vi "FIU card.vi"(8 "error in (no error)":errorcluster, 11 "Node Ptr":T3 format="%.0x") -> (0 "error out":errorcluster)   [LabVIEW 2013, in "SLSC configuration System Explorer.lvlib"]
uses:
  SLSC configuration System Explorer.lvlib
  <vilib>/NI Veristand/Custom Device API/Custom Device Item Ref.ctl
  Shared/Card Postion.ctl
  Shared/Constants.vi
  <vilib>/NI Veristand/Custom Device API/Get Item Property (U16).vi
  <vilib>/NI Veristand/Custom Device API/Set Item Property (Variant).vi
  <vilib>/NI Veristand/Custom Device API/Custom Device API.lvlib
  Shared/SLSC configuration Shared.lvlib
panel:
  in  "Card Position":T1
  in  "Fault 8":T2(ring)
  in  "Fault 7":T2(ring)
  in  "Fault 6":T2(ring)
  in  "Fault 5":T2(ring)
  in  "Fault 4":T2(ring)
  in  "Fault 3":T2(ring)
  in  "Fault 2":T2(ring)
  in  "Header 2":cluster{"Section Name":string}={"Section Name"="FIU Initial Configuration"}
  in  "Fault 1":T2(ring)
  in  "Header":cluster{"Section Name":string}={"Section Name"="FIU Card Settings"}
  in  "Description":string
  in  "Name":string
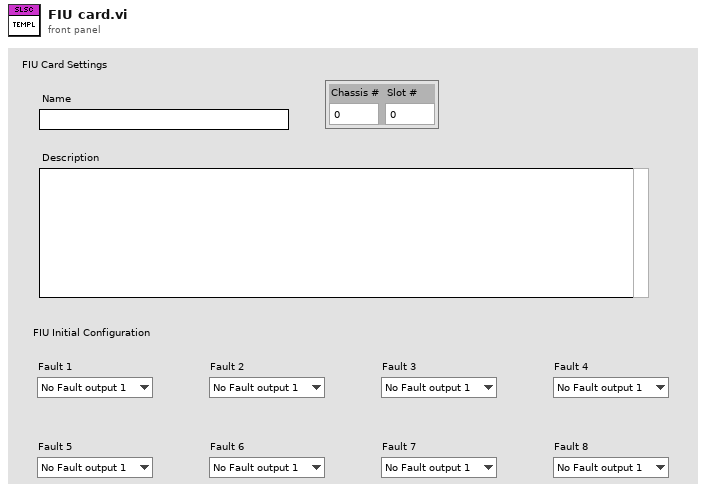
[diagram p1: front panel]
types:
  T1 = typedef "SLSC configuration Shared.lvlib/Card Postion.ctl" = cluster{"Chassis #":u8, "Slot #":u8}
  T2 = enum16{"No Fault output 1", "Open Ckt 100Hz", "Ground 100Hz", "Open Circuit", "Ground", "Rail 1", "Rail 2", "No Fault output 2"}
  T3 = typedef "Custom Device API.lvlib/Custom Device Item Ref.ctl" = u64
  T4 = typedef "Custom Device API.lvlib/Custom Device Commands.ctl" = enum16{"Default", "Item renamed", "Shutdown", "Dynamic button pressed"}
  T5 = typedef "Custom Device API.lvlib/Custom Device Item Info.ctl" = cluster{"Name":string, "Is Channel":bool, "GUID":string, "Is Waveform":bool}
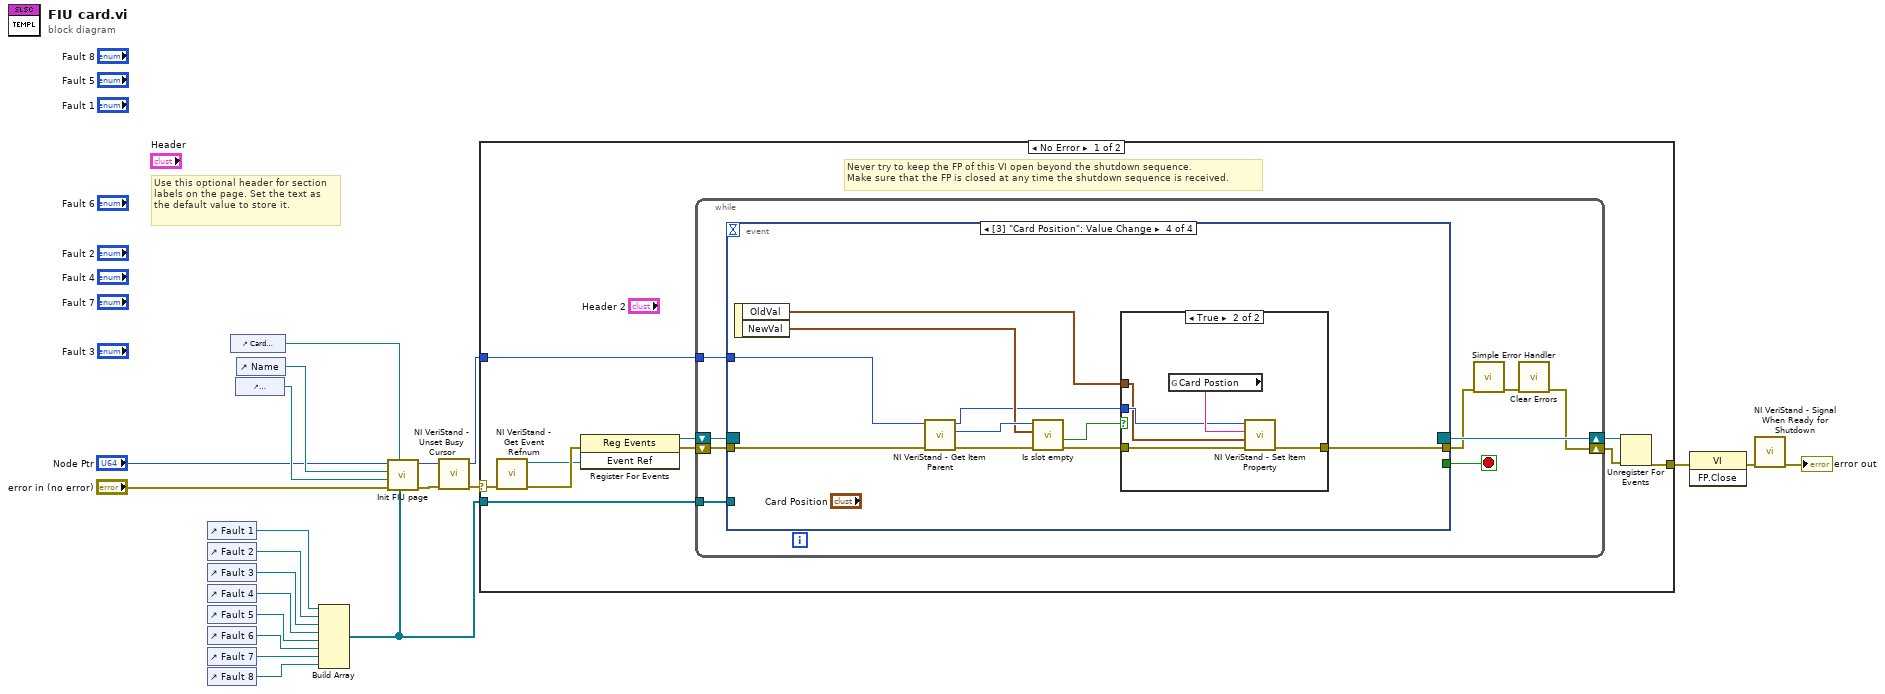
[diagram p0: block diagram]
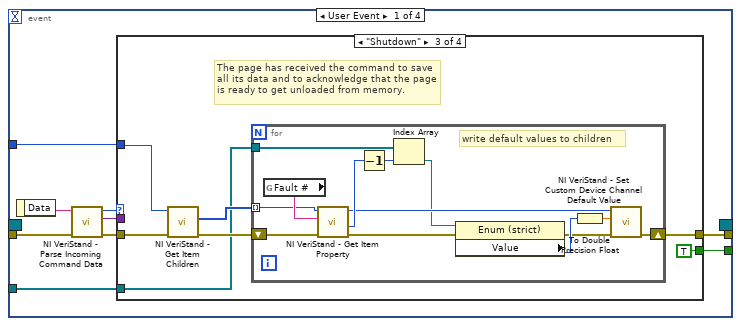
[diagram p2: hidden frame]
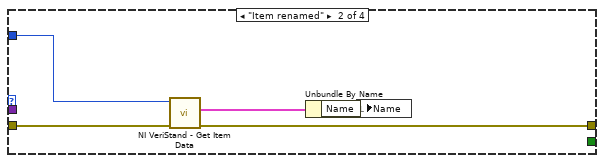
[diagram p4: hidden frame]
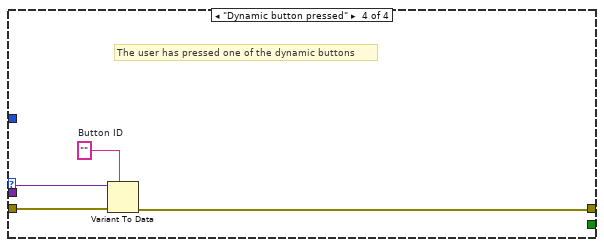
[diagram p5: hidden frame]
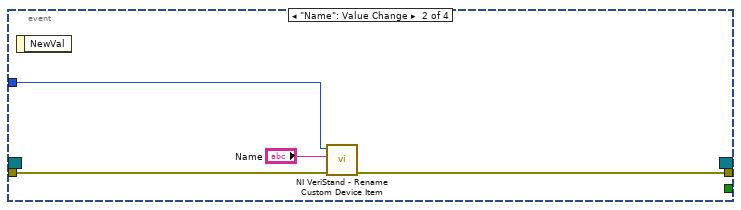
[diagram p6: hidden frame]
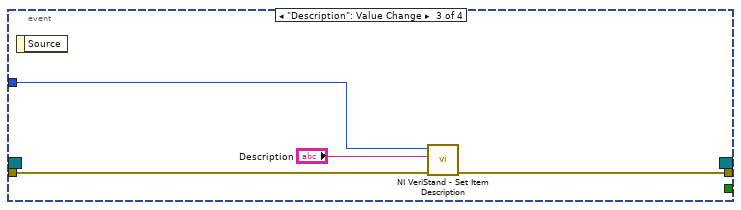
[diagram p7: hidden frame]
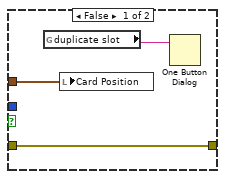
[diagram p8: hidden frame]
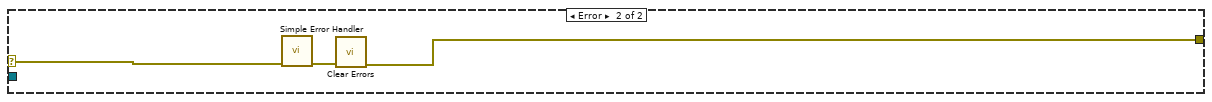
[diagram p9: hidden frame]
diagram:
  # "Use this optional header for section labels on the page. Set the text as the default value to store it."
  n1 = control-ref of="Fault 1"() -> (w13:refnum<vi>)
  n2 = control-ref of="Fault 2"() -> (w12:refnum<vi>)
  n3 = control-ref of="Fault 3"() -> (w11:refnum<vi>)
  n4 = control-ref of="Fault 4"() -> (w10:refnum<vi>)
  n5 = control-ref of="Fault 5"() -> (w9:refnum<vi>)
  n6 = control-ref of="Fault 6"() -> (w8:refnum<vi>)
  n7 = control-ref of="Fault 7"() -> (w7:refnum<vi>)
  n8 = control-ref of="Fault 8"() -> (w6:refnum<vi>)
  n9 = control-ref of="Card Position"() -> (w1:refnum<vi>)
  n10 = control-ref of="Description"() -> (w4:refnum<vi>)
  n11 = control-ref of="Name"() -> (w5:refnum<vi>)
  n12 = Build Array(w13, w12, w11, w10, w9, w8, w7, w6) -> (w2:refnum<vi>[])
  n13 = call "Init FIU page.vi"("Fault controls"=w2, "Card Position"=w1, "error in (no error)"="error in (no error)", "Description"=w4, "Name"=w5, "Node Ptr"="Node Ptr") -> ("error out"=w17:errorcluster, "Node Ptr out"=w14:T3)  [unwired: 4 in]
  n14 = call <vilib>:"NI VeriStand - Unset Busy Cursor.vi"("error in (no error)"=w17) -> ("error out"=w16:errorcluster)  [unwired: 10 out]
  n15 = case shown="No Error" w16 {
    selector: w16 -> [w22 w107]
    tunnel: [w27 w105] -> w20
    tunnel: w14 -> [w23 _]
    tunnel: w2 -> [w21 _]
    frame No Error {
      # "Never try to keep the FP of this VI open beyond the shutdown sequence.\nMake sure that the FP is closed at any time the shutdown sequence is received."
      n16 = call <vilib>:"NI VeriStand - Get Event Refnum.vi"("error in (no error)"=w22) -> ("error out"=w30:errorcluster, "Event Ref"=w26:refnum<user-event>)  [unwired: 9 out]
      n17 = register-events(error in=w30, w26) -> (reference out=w24:refnum<event-registration>, error out=w25:errorcluster)  [unwired: 1 in]
      n18 = while {
        tunnel: w23 -> [w35]
        shift-right: [w32] -> w28
        shift-left: w25 -> [w38]
        shift-right: [w39] -> w29
        shift-left: w24 -> [w37]
        tunnel: w21 -> [w31]
        stop <- w36 stop-if-true
        n19 = event shown="[3] \"Card Position\": Value Change" {
          selector: w37 -> [_ _ _ _]
          dyn-events: [_ _ _ _] -> w39
          timeout: _ -> [_ _ _ _]
          tunnel: w38 -> [w48 w82 w85 w88]
          tunnel: [w44 _ _ _] -> w36
          tunnel: [w43 w81 w84 w94] -> w34
          tunnel: w35 -> [w42 w80 w86 w93]
          tunnel: w31 -> [w40 _ _ _]
          event User Event {
            n20 = event-data() -> ("Data"=w47:string)  [unwired: 1 out]
            n21 = call <vilib>:"NI VeriStand - Parse Incoming Command Data.vi"("error in (no error)"=w48, "Incoming data"=w47) -> ("error out"=w46:errorcluster, "Outgoing data"=w41:variant, "Action"=w45:T4)  [unwired: 7 out]
            n22 = case shown="\"Shutdown\"" w45 {
              tunnel: w46 -> [w49 w54 w58 w78]
              tunnel: [_ _ TRUE _] -> w44
              tunnel: [w49 w51 w60 w75] -> w43
              tunnel: w42 -> [_ w53 w56 _]
              tunnel: w41 -> [_ _ _ w77]
              tunnel: w40 -> [_ _ w55 _]
              frame "Default", Default {
              }
              frame "Item renamed" {
                n23 = call <vilib>:"NI VeriStand - Get Item Data.vi"("error in (no error)"=w54, "Item Ref in"=w53) -> ("error out"=w51:errorcluster, "Item Info"=w52:T5)  [unwired: 8 out]
                n24 = Unbundle By Name(w52) -> ("Name"=w50:string)
                n25 = local write "Name"(w50) -> ()
              }
              frame "Shutdown" {
                # "The page has received the command to save all its data and to acknowledge that the page is ready to get unloaded from memory."
                n26 = call <vilib>:"NI VeriStand - Get Item Children.vi"("error in (no error)"=w58, "Item Ref in"=w56) -> ("error out"=w57:errorcluster, "Child Refs"=w59:T3[])  [unwired: 6 in, 2 out]
                n27 = for {
                  shift-right: [w70] -> w60
                  shift-left: w57 -> [w73]
                  tunnel: w59 -> [w64] mode=indexing
                  tunnel: w55 -> [w63]
                  # "write default values to children"
                  n28 = global read "Constants.vi" "Fault #"() -> (w74:string)
                  n29 = call-poly <vilib>:"NI VeriStand - Get Item Property.vi"("error in (no error)"=w73, "Property Name"=w74, "Item Ref in"=w64) -> ("error out"=w67:errorcluster, "Value"=w72:u16, "Item Ref out"=w69:T3)  [unwired: 5 in, 1 out]
                  n30 = Decrement(x=w72) -> (x-1=w71:u16)
                  n31 = Index Array(array=w63, index=w71) -> (element=w62:refnum<vi>)
                  n32 = property class="Enum (strict)"(reference=w62, error in=w67) -> (error out=w65:errorcluster, "Value"=w66:T2)  [unwired: 1 out]
                  n33 = To Double Precision Float(number=w66) -> (double precision float=w68:dbl)
                  n34 = call <vilib>:"NI VeriStand - Set Custom Device Channel Default Value.vi"("error in (no error)"=w65, "Default Value"=w68, "Channel Ref in"=w69) -> ("error out"=w70:errorcluster)  [unwired: 7 in, 1 out]
                }
              }
              frame "Dynamic button pressed" {
                w76 = ""  # Button ID
                # "The user has pressed one of the dynamic buttons"
                n35 = Variant To Data(error in=w78, type=w76, Variant=w77) -> (error out=w75:errorcluster)  [unwired: 1 out]
              }
            }
          }
          event "Name": Value Change {
            n36 = event-data() -> ()  [unwired: 2 out]
            n37 = call <vilib>:"NI VeriStand - Rename Custom Device Item.vi"("error in (no error)"=w82, "New Name"="Name", "Item Ref in"=w80) -> ("error out"=w81:errorcluster)  [unwired: 1 in, 7 out]
          }
          event "Description": Value Change {
            n38 = event-data() -> ()  [unwired: 2 out]
            n39 = call <vilib>:"NI VeriStand - Set Item Description.vi"("error in (no error)"=w85, "Description"="Description", "Item Ref in"=w86) -> ("error out"=w84:errorcluster)  [unwired: 8 out]
          }
          event Value Change {
            n40 = event-data() -> ("OldVal"=w87:T1, "NewVal"=w91:T1)  [unwired: 1 out]
            n41 = call <vilib>:"NI VeriStand - Get Item Parent.vi"("error in (no error)"=w88, "Item Ref in"=w93) -> ("error out"=w90:errorcluster, "Parent Ref"=w92:T3, "Item Ref out"=w89:T3)  [unwired: 6 in, 1 out]
            n42 = call "Is slot empty.vi"("error in (no error)"=w90, "Card Position"=w91, "Node Ptr"=w92) -> ("error out"=w96:errorcluster, "Empty?"=w95:bool)  [unwired: 6 in, 1 out]
            n43 = case shown="True" w95 {
              tunnel: w96 -> [w98 w101]
              tunnel: [w98 w103] -> w94
              tunnel: w89 -> [_ w102]
              tunnel: w87 -> [w97 w100]
              frame False {
                n44 = global read "Constants.vi" "duplicate slot"() -> (w99:string)
                n45 = local write "Card Position"(w97) -> ()
                n46 = One Button Dialog(message=w99) -> ()  [unwired: 1 in, 1 out]
              }
              frame True {
                n47 = global read "Constants.vi" "Card Postion"() -> (w104:string)
                n48 = call-poly <vilib>:"NI VeriStand - Set Item Property.vi"("error in (no error)"=w101, "Value"=w100, "Property Name"=w104, "Item Ref in"=w102) -> ("error out"=w103:errorcluster)  [unwired: 5 in, 2 out]
              }
            }
          }
        }
        n49 = call <vilib>:"Simple Error Handler.vi"("error in (no error)"=w34) -> ("error out"=w33:errorcluster)  [unwired: 1 in, 7 out]
        n50 = call <vilib>:"Clear Errors.vi"("error in (no error)"=w33) -> ("error out"=w32:errorcluster)  [unwired: 6 out]
      }
      n51 = Unregister For Events(event registration refnum=w29, error in=w28) -> (error out=w27:errorcluster)
    }
    frame Error {
      n52 = call <vilib>:"Simple Error Handler.vi"("error in (no error)"=w107) -> ("error out"=w106:errorcluster)  [unwired: 1 in, 7 out]
      n53 = call <vilib>:"Clear Errors.vi"("error in (no error)"=w106) -> ("error out"=w105:errorcluster)  [unwired: 6 out]
    }
  }
  n54 = invoke class="VI" method="FP.Close"(error in=w20) -> (error out=w19:errorcluster)  [unwired: 2 in, 2 out]
  n55 = call <vilib>:"NI VeriStand - Signal When Ready for Shutdown.vi"("error in (no error)"=w19) -> ("error out"=→"error out":errorcluster)  [unwired: 10 out]
